vi "visionAlgorithm.vi"(7 "error in":errorcluster) -> (27 "error out":errorcluster)   [LabVIEW 2019]
uses:
  <vilib>/vision/Image Controls.llb/IMAQ Image.ctl
panel:
  out "Error Out":errorcluster
  in  "Range":cluster{"Lower value":sgl, "Upper value":sgl}={"Lower value"=67.0, "Upper value"=255.0}
  out "Image Out 2":T1
  out "Image Out":T1(plugin-control)
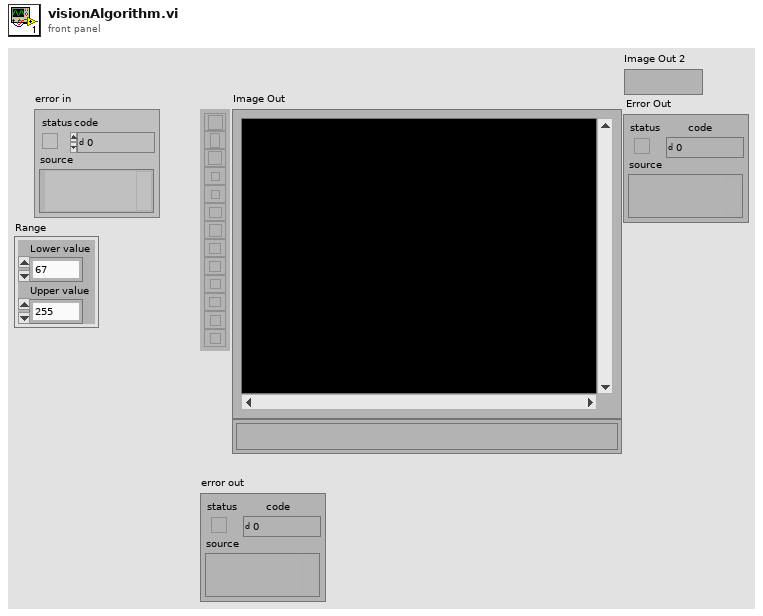
[diagram p1: front panel]
types:
  T1 = typedef "IMAQ Image.ctl" = refnum<image>
  T2 = typedef "Image Type" = u32
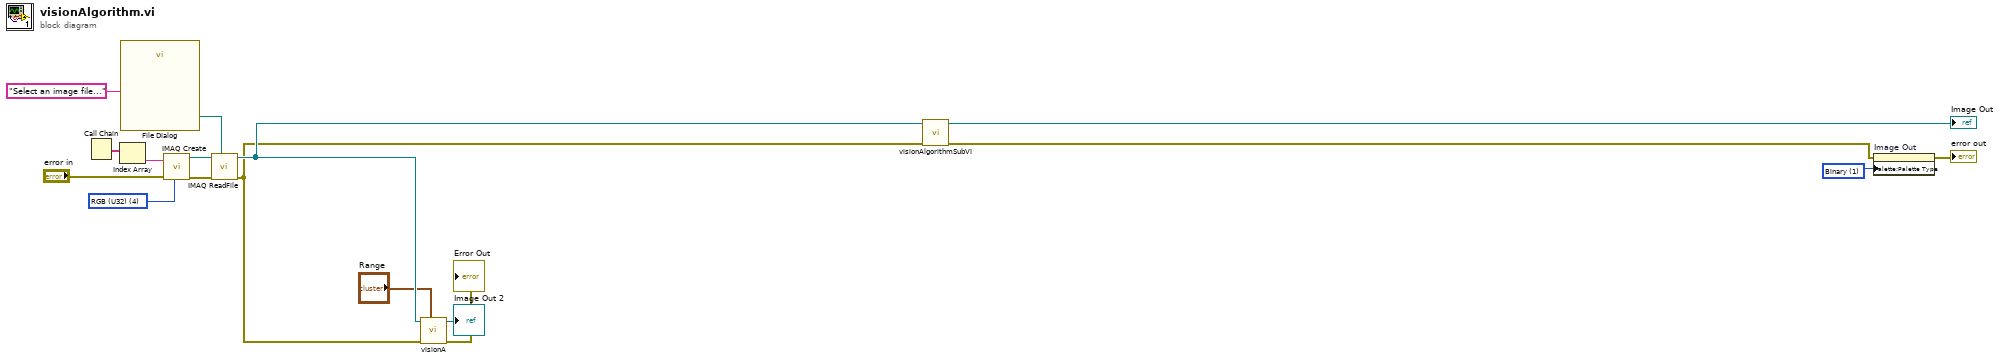
[diagram p0: block diagram]
diagram:
  w6 = u32 1 items=["Grayscale", "Binary", "Gradient", "Rainbow", "Temperature", "User Defined", "Binary 16 Bit", "Gradient 16 Bit", "Rainbow 16 Bit", "Temperature 16 Bit", "User Defined 16 Bit"] ("Palette Type")
  w10 = T2 4 items=["Grayscale (U8)", "Grayscale (I16)", "Grayscale (SGL)", "Complex (CSG)", "RGB (U32)", "HSL (U32)", "RGB (U64)", "Grayscale (U16)"] ("Image Type")
  n1 = Call Chain() -> (call chain=w14:string[])
  n2 = Index Array(array=w14) -> (element=w13:string)  [unwired: 1 in]
  n3 = call "File Dialog"("prompt"="Select an image file...") -> ("selected path"=w11:path)  [unwired: 6 in, 8 out]
  n4 = call "IMAQ Create"("Image Name"=w13, "Image Type"=w10, "error in (no error)"="error in") -> ("New Image"=w17:T1, "error out"=w16:errorcluster)  [unwired: 1 in, 1 out]
  n5 = call "IMAQ ReadFile"("File Path"=w11, "error in (no error)"=w16, "Image"=w17) -> ("error out"=w4:errorcluster, "Image Out"=w5:T1)  [unwired: 2 in, 5 out]
  n6 = call "visionA.vi"("Range"="Range", "Error In"=w4, "Image In"=w5) -> ("Error Out"=→"Error Out":errorcluster, "Image Out"=→"Image Out 2":T1)  [unwired: 7 in]
  n7 = call "visionAlgorithmSubVI.vi"("error in (no error)"=w4, "Refnum in"=w5) -> ("error out"=w9:errorcluster, "Refnum out"=→"Image Out":T1)  [unwired: 5 in, 3 out]
  n8 = property on="Image Out" class="ImageControl"(error in=w9, "Palette:Palette Type"=w6) -> (error out=→"error out":errorcluster)  [unwired: 1 in, 1 out]
